vi "Build Stim Init Cmd_v0.vi"(0 "Stimulator In":T2={"Log File In"=refnum, "Stimulator In"="", "Stimulator Mode"="", "Log Data"=FALSE, "Doublet/Triplet  Interval"=0.0, "Stim Frequency"=40.0, "N-Factor"=0, "Active Channels"=[FALSE, FALSE, FALSE, FALSE, FALSE], "Low-Frequency Channels"=[FALSE, FALSE, FALSE, FALSE, FALSE], "Stimulator State"=enum."Closed", "Mode Array"=[], "Current Array"=[], "Pulse Duration Array"=[], "VISA Timeout"=50}) -> (2 "Stimulator Out":T2={"Log File In"=refnum, "Stimulator In"="", "Stimulator Mode"="", "Log Data"=FALSE, "Doublet/Triplet  Interval"=0.0, "Stim Frequency"=40.0, "N-Factor"=0, "Active Channels"=[FALSE, FALSE, FALSE, FALSE, FALSE], "Low-Frequency Channels"=[FALSE, FALSE, FALSE, FALSE, FALSE], "Stimulator State"=enum."Closed", "Mode Array"=[], "Current Array"=[], "Pulse Duration Array"=[], "VISA Timeout"=50}, 3 "Command":T1)   [LabVIEW 2019]
uses:
  Controls/Stimulator Cluster.ctl
  Controls/Stimulator Mode.ctl
  Version 2/Data Type Defs/Pulse Mode (array).ctl
  Controls/Stim Current Array.ctl
  Controls/Pulse Duration Array.ctl
  NumArray to CatStr.vi
  Archive/StrArray to CatStr.vi
panel:
  out "N-Factor":u8
  out "Interpulse Interval (ms)":dbl
  out "Channel LF Boolean Array":bool[](array[boolean])
  out "Channel Stim Boolean Array":bool[](array[boolean])=[TRUE, TRUE, TRUE, TRUE, TRUE]
  out "Stim Frequency (Hz)":dbl=40.0
  # "Inputs\nStim Frequency - the main frequency of stimulation in Hz.  The Hasomed Rehastim Science Mode documentation defines this as 1/t1.  We typically use 40 Hz for FES applications.\nGroup Time - for multi-pulse stimulation, enter the inter-pulse interval (aka pulse repetition interval) here.  We typically use single pulses (Group Time = 0).\nN factor - the factor by which t1 is multiplied to get the \"Low Frequency\" channel period.  This is optional - we typically do not use it.\nChannel Stim Boolean Array - defines the active channels (up to 8).\nChannel LF Boolean Array - defines the channels for which \"low frequency\" will be used.  Low frequency is defined as 1/(N_factor * Stim_Frequency).\n\nOutputs\nChannel List Mode Init Cmd String - the string of Hex numbers representing the final command."
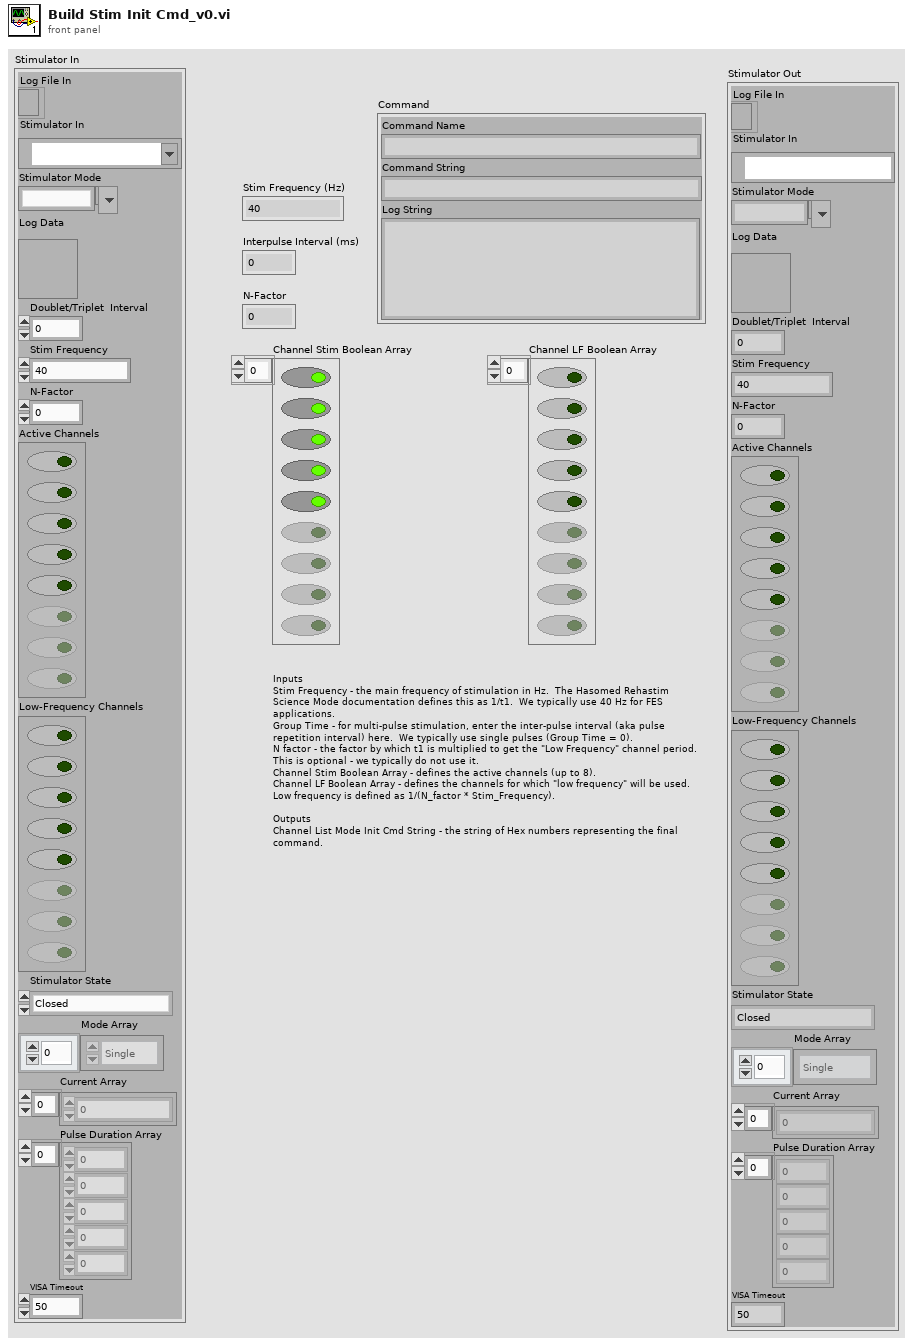
[diagram p1: front panel]
types:
  T1 = cluster{"Command Name":string, "Command String":string, "Log String":string}
  T2 = typedef "Stimulator Cluster.ctl" = cluster{"Log File In":refnum<file>, "Stimulator In":refnum<visa-resource-name>, "Stimulator Mode":T3, "Log Data":bool, "Doublet/Triplet  Interval":dbl, "Stim Frequency":dbl, "N-Factor":u8, "Active Channels":bool[], "Low-Frequency Channels":bool[], "Stimulator State":enum16{"Closed", "Open", "Initialized", "Stimulating"}, "Mode Array":T4, "Current Array":T5, "Pulse Duration Array":T6, "VISA Timeout":u32}
  T3 = typedef "Stimulator Mode.ctl" = string
  T4 = typedef "Pulse Mode (array).ctl" = enum16{"Single", "Doublet", "Triplet"}[]
  T5 = typedef "Stim Current Array.ctl" = u8[]
  T6 = typedef "Pulse Duration Array.ctl" = u32[]
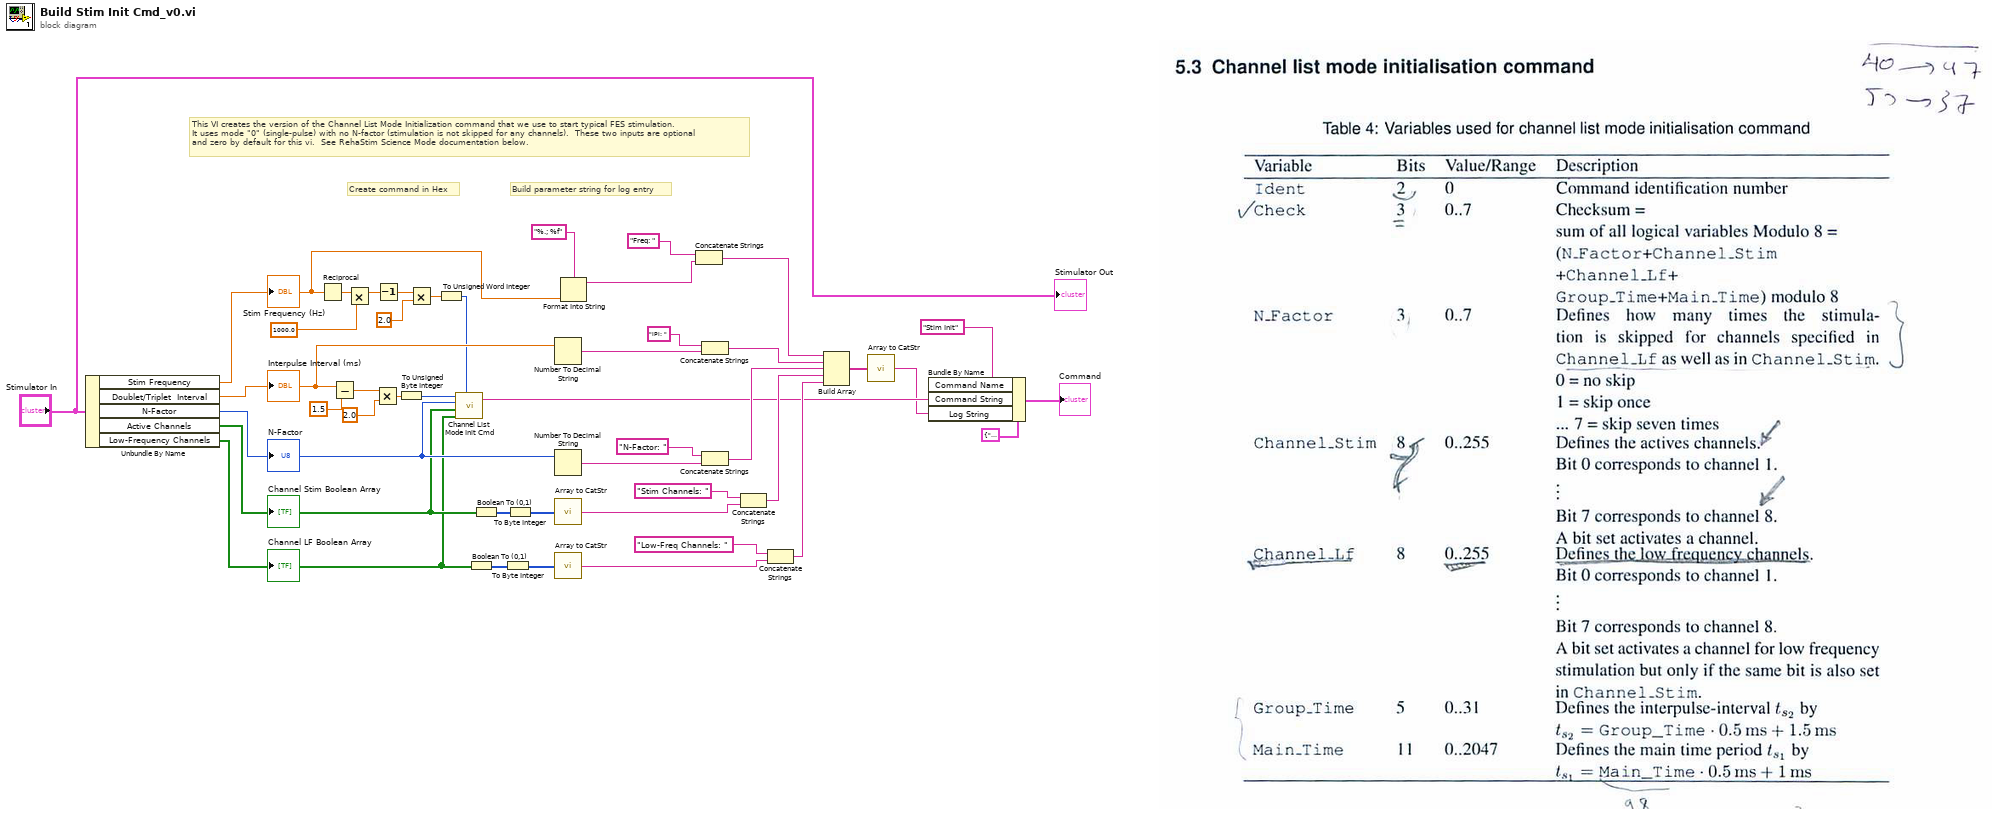
[diagram p0: block diagram]
diagram:
  # "Build parameter string for log entry"
  # "Create command in Hex"
  # "This VI creates the version of the Channel List Mode Initialization command that we use to start typical FES stimulation.\nIt uses mode \"0\" (single-pulse) with no N-factor (stimulation is not skipped for any channels).  These two inputs are optional\nand zero by default for this vi.  See RehaStim Science Mode documentation below."
  n1 = Unbundle By Name("Stimulator In") -> ("Stim Frequency"=w10:dbl, "Doublet/Triplet  Interval"=w15:dbl, "N-Factor"=w14:u8, "Active Channels"=w13:bool[], "Low-Frequency Channels"=w12:bool[])
  "Stim Frequency (Hz)" <- w10
  "Channel Stim Boolean Array" <- w13
  "Channel LF Boolean Array" <- w12
  "Interpulse Interval (ms)" <- w15
  "N-Factor" <- w14
  n2 = Reciprocal(x=w10) -> (1/x=w44:dbl)
  n3 = Subtract(x=w15, y=1.5) -> (x-y=w38:dbl)
  n4 = Multiply(x=w44, y=1000.0) -> (x*y=w41:dbl)
  n5 = Multiply(x=w38, y=2.0) -> (x*y=w36:dbl)
  n6 = Decrement(x=w41) -> (x-1=w43:dbl)
  n7 = To Unsigned Byte Integer(number=w36) -> (unsigned 8bit integer=w1:u8)
  n8 = Multiply(x=w43, y=2.0) -> (x*y=w35:dbl)
  n9 = To Unsigned Word Integer(number=w35) -> (unsigned 16bit integer=w2:u16)
  n10 = call "Channel List Mode Init Cmd.vi"("Main time"=w2, "Channel LF Boolean Array"=w12, "Channel Stim Boolean Array"=w13, "N factor"=w14, "Group Time"=w1) -> ("Channel List Mode Init Cmd String"=w5:string)  [unwired: 2 in]
  n11 = Boolean To (0,1)(Boolean=w12) -> (0, 1=w31:i16[])
  n12 = Boolean To (0,1)(Boolean=w13) -> (0, 1=w33:i16[])
  n13 = To Byte Integer(number=w31) -> (8bit integer=w30:i8[])
  n14 = To Byte Integer(number=w33) -> (8bit integer=w32:i8[])
  n15 = Number To Decimal String(number=w15) -> (decimal integer string=w26:string)  [unwired: 1 in]
  n16 = Number To Decimal String(number=w14) -> (decimal integer string=w23:string)  [unwired: 1 in]
  n17 = call-poly "Array to CatStr.vi"("Array"=w32) -> ("spreadsheet string"=w21:string)
  n18 = call-poly "Array to CatStr.vi"("Array"=w30) -> ("spreadsheet string"=w19:string)
  n19 = Format Into String(format string="%.; %f", w10) -> (resulting string=w8:string)  [unwired: 2 in, 1 out]
  n20 = Concatenate Strings("Freq: " ("string"), w8) -> (w28:string)
  n21 = Concatenate Strings("IPI: " ("string"), w26) -> (w25:string)
  n22 = Concatenate Strings("N-Factor: " ("string"), w23) -> (w18:string)
  n23 = Concatenate Strings("Stim Channels: " ("string"), w21) -> (w17:string)
  n24 = Concatenate Strings("Low-Freq Channels: " ("string"), w19) -> (w16:string)
  n25 = Build Array(w28, w25, w18, w17, w16) -> (w34:string[])
  n26 = call-poly "Array to CatStr.vi"("String Array"=w34) -> ("spreadsheet string"=w4:string)
  n27 = Bundle By Name(cluster=T1 {"Command Name"="", "Command String"="", "Log String"=""}, "Command Name"="Stim Init", "Command String"=w5, "Log String"=w4) -> (→"Command":T1)
  "Stimulator Out" <- "Stimulator In"
